vi "Create Message Data Clusters (complex).vi"(8 "error in (no error)":errorcluster, 10 "Message Metadata":T1, 11 "LVClassLibrary in":refnum<vi>) -> (0 "error out":errorcluster, 3 "LVClassLibrary out":refnum<vi>)   [LabVIEW 2019, in "gRPC Scripting Tools.lvlib"]
uses:
  gRPC Scripting Tools.lvlib
  TypeDefs/Message Metadata (Scripting).ctl
  TypeDefs/Message Element Metadata (Scripting).ctl
  gRPC interface/Server API/typeDefs/Message Element Type.ctl
  gRPC interface/gprc-lvsupport.lvlib
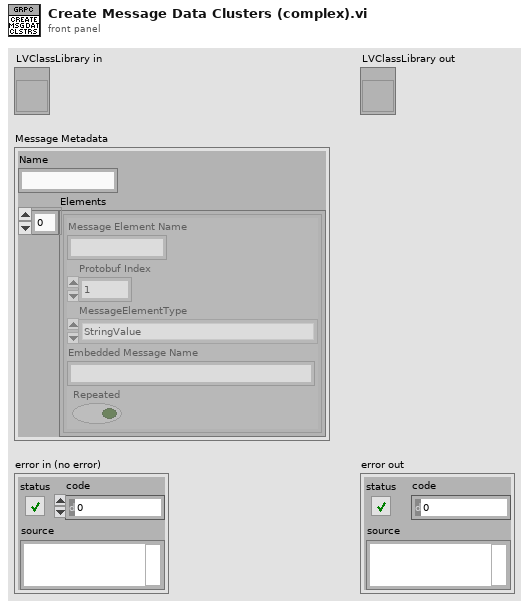
[diagram p1: front panel]
types:
  T1 = typedef "gRPC Scripting Tools.lvlib/Message Metadata (Scripting).ctl" = cluster{"Name":string, "Elements":T2[]}
  T2 = typedef "gRPC Scripting Tools.lvlib/Message Element Metadata (Scripting).ctl" = cluster{"Message Element Name":string, "Protobuf Index":i32, "MessageElementType":T3, "Embedded Message Name":string, "Repeated":bool}
  T3 = typedef "gprc-lvsupport.lvlib/Message Element Type.ctl" = enum32{"Int32Value", "FloatValue", "DoubleValue", "BoolValue", "StringValue", "MessageValue", ""}
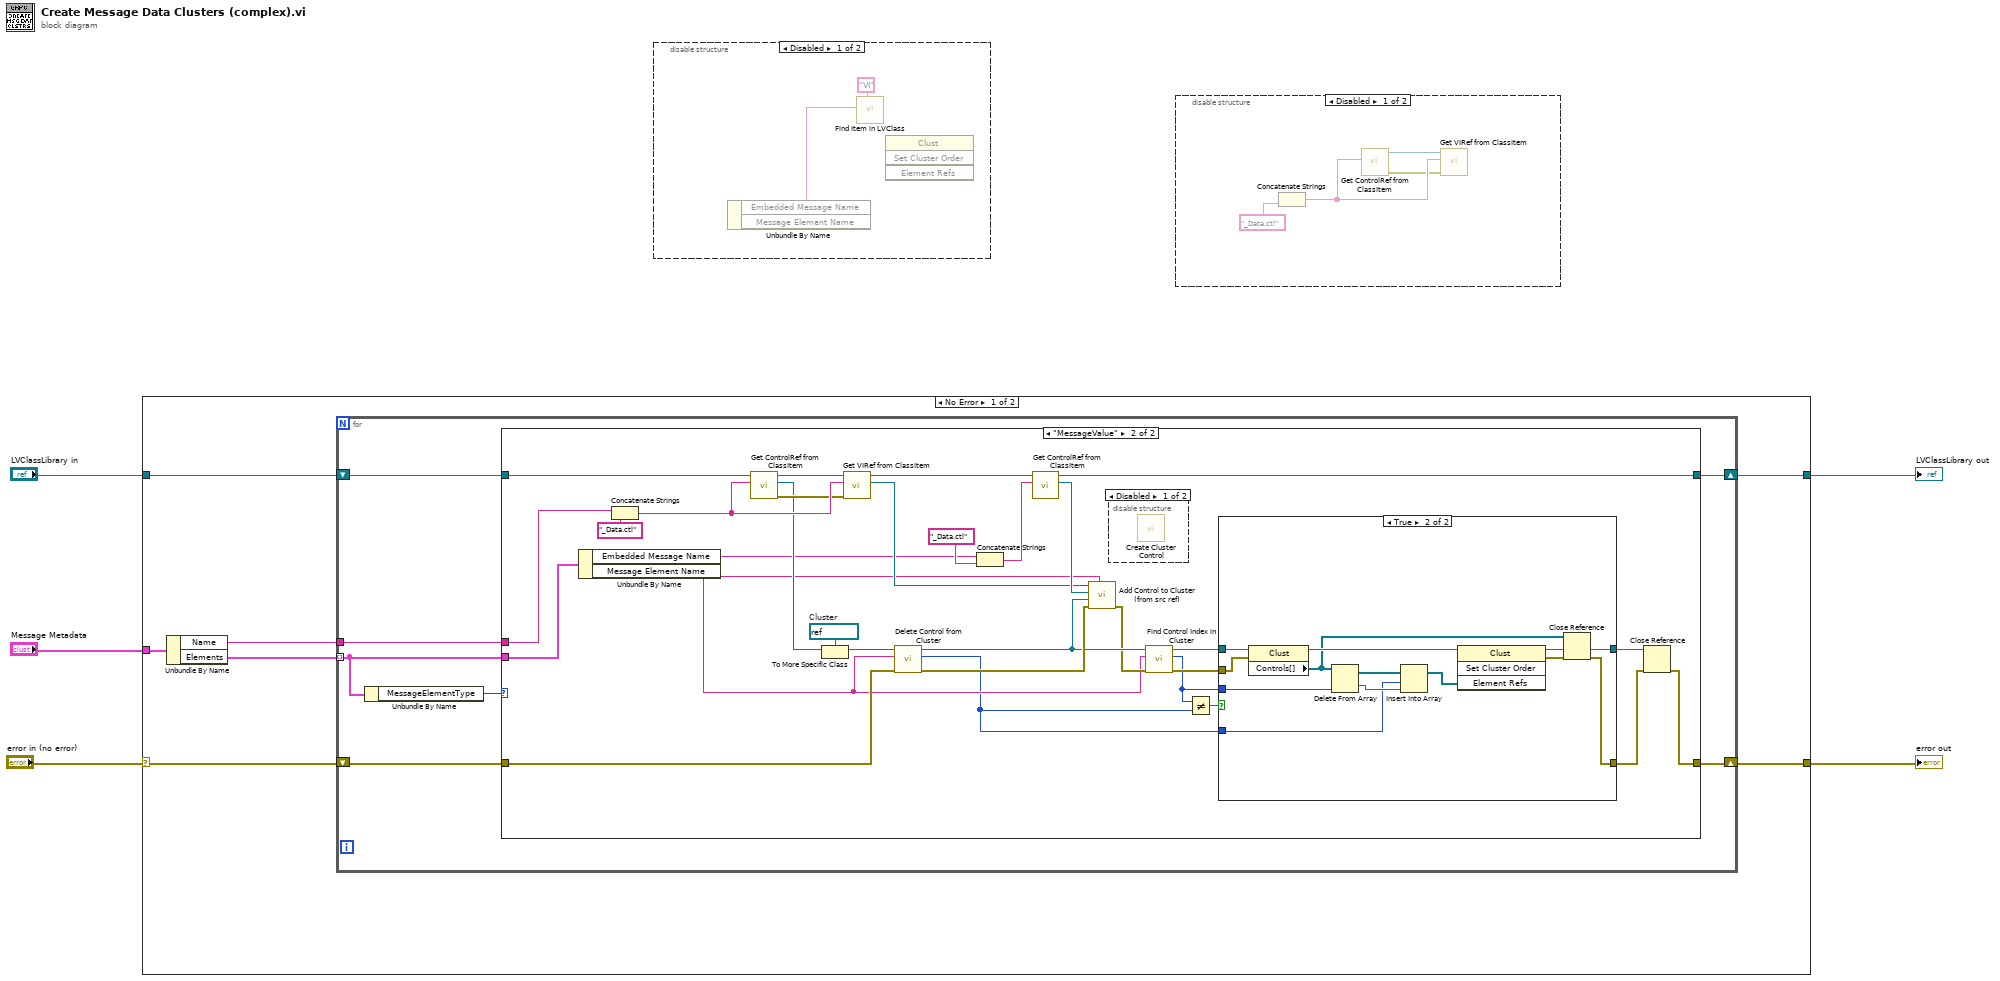
[diagram p0: block diagram]
diagram:
  n1 = case shown="No Error" "error in (no error)" {
    selector: "error in (no error)" -> [w7 w66]
    tunnel: "Message Metadata" -> [w12 _]
    tunnel: "LVClassLibrary in" -> [w8 w67]
    tunnel: [w9 w66] -> w3
    tunnel: [w10 w67] -> w2
    frame No Error {
      n2 = Unbundle By Name(w12) -> ("Name"=w6:string, "Elements"=w11:T2[])
      n3 = for {
        tunnel: w11 -> [w16] mode=indexing
        shift-right: [w17] -> w10
        shift-left: w8 -> [w18]
        shift-right: [w13] -> w9
        shift-left: w7 -> [w14]
        tunnel: w6 -> [w15]
        n4 = Unbundle By Name(w16) -> ("MessageElementType"=w19:T3)
        n5 = case shown="\"MessageValue\"" w19 {
          tunnel: w16 -> [_ w35]
          tunnel: w18 -> [w21 w42]
          tunnel: [w21 w48] -> w17
          tunnel: w15 -> [_ w40]
          tunnel: w14 -> [w20 w33]
          tunnel: [w20 w23] -> w13
          frame "", Default {
          }
          frame "MessageValue" {
            w37 = refnum<vi> refnum  # Cluster
            n6 = Unbundle By Name(w35) -> ("Embedded Message Name"=w34:string, "Message Element Name"=w30:string)
            n7 = Concatenate Strings(w40, "_Data.ctl" ("string")) -> (w44:string)
            n8 = call "Get ControlRef from ClassItem.vi"("Item Name"=w44, "LVClassLibrary in"=w42) -> ("error out"=w43:errorcluster, "Control ref out"=w38:refnum<vi>, "LVClassLibrary out"=w45:refnum<vi>)  [unwired: 6 in, 1 out]
            n9 = To More Specific Class(target class=w37, reference=w38) -> (specific class reference=w36:refnum<vi>)  [unwired: 1 in, 1 out]
            n10 = call "Get VIRef from ClassItem.vi"("error in (no error)"=w43, "Item Name"=w44, "LVClassLibrary in"=w45) -> ("VIref out"=w39:refnum<vi>, "LVClassLibrary out"=w41:refnum<vi>)  [unwired: 5 in, 2 out]
            n11 = call "Delete Control from Cluster.vi"("error in (no error)"=w33, "Control Name in"=w30, "Cluster ref in"=w36) -> ("error out"=w47:errorcluster, "Deleted Index"=w25:i32, "Cluster ref out"=w32:refnum<vi>)  [unwired: 6 in]
            n12 = Concatenate Strings(w34, "_Data.ctl" ("string")) -> (w50:string)
            n13 = call "Get ControlRef from ClassItem.vi"("Item Name"=w50, "LVClassLibrary in"=w41) -> ("Control ref out"=w49:refnum<vi>, "LVClassLibrary out"=w48:refnum<vi>)  [unwired: 6 in, 2 out]
            n14 = call "Add Control to Cluster (from src ref).vi"("New Control Label"=w30, "error in (no error)"=w47, "Cluster ref in (owner)"=w32, "Control ref in"=w49, "Owning VI ref in"=w39) -> ("error out"=w31:errorcluster)  [unwired: 3 in, 3 out]
            n15 = disable-structure shown="Disabled" {
              frame Disabled {
                n16 = call "Create Cluster Control.vi"() -> ()  [unwired: 9 in, 3 out]
              }
              frame Enabled {
              }
            }
            n17 = call "Find Control Index in Cluster.vi"("error in (no error)"=w31, "Control Name"=w30, "Cluster ref in"=w32) -> ("error out"=w27:errorcluster, "Control Index"=w26:i32, "Cluster ref out"=w28:refnum<vi>)  [unwired: 6 in]
            n18 = Not Equal?(x=w26, y=w25) -> (x != y?=w29:bool)
            n19 = case shown="True" w29 {
              tunnel: w28 -> [w52 w65]
              tunnel: w27 -> [w53 w64]
              tunnel: w26 -> [_ w63]
              tunnel: w25 -> [_ w60]
              tunnel: [w53 w55] -> w24
              tunnel: [w52 w54] -> w22
              frame False {
              }
              frame True {
                n20 = property class="Clust"(reference=w65, error in=w64) -> (reference out=w59:refnum<vi>, "Controls[]"=w56:refnum<vi>[])  [unwired: 1 out]
                n21 = Delete From Array(array=w56, index=w63) -> (deleted portion=w61:refnum<vi>, array with subset deleted=w62:refnum<vi>[])  [unwired: 1 in]
                n22 = Insert Into Array(array=w62, index=w60, new element=w61) -> (w58:refnum<vi>[])
                n23 = invoke class="Clust" method="Set Cluster Order"(reference=w59, "Element Refs"=w58) -> (reference out=w54:refnum<vi>, error out=w57:errorcluster)  [unwired: 2 in, 2 out]
                n24 = Close Reference(reference=w56, error in (no error)=w57) -> (error out=w55:errorcluster)
              }
            }
            n25 = Close Reference(reference=w22, error in (no error)=w24) -> (error out=w23:errorcluster)
          }
        }
      }
    }
    frame Error {
    }
  }
  "error out" <- w3
  "LVClassLibrary out" <- w2
  n26 = disable-structure shown="Disabled" {
    frame Disabled {
      n27 = Unbundle By Name() -> ("Embedded Message Name"=w69:string)  [unwired: 1 in, 1 out]
      n28 = call "Find Item in LVClass.vi"("Item Type"="VI", "Item Name"=w69) -> ()  [unwired: 6 in, 4 out]
      n29 = invoke class="Clust" method="Set Cluster Order"() -> ()  [unwired: 4 in, 4 out]
    }
    frame Enabled {
    }
  }
  n30 = disable-structure shown="Disabled" {
    frame Disabled {
      n31 = Concatenate Strings("_Data.ctl" ("string")) -> (w71:string, w75:string)
      n32 = call "Get ControlRef from ClassItem.vi"("Item Name"=w71) -> ("error out"=w70:errorcluster, "Control ref out"=w73:refnum<vi>, "LVClassLibrary out"=w72:refnum<vi>)  [unwired: 7 in, 1 out]
      n33 = call "Get VIRef from ClassItem.vi"("error in (no error)"=w70, "Item Name"=w71, "LVClassLibrary in"=w72) -> ()  [unwired: 5 in, 4 out]
    }
    frame Enabled {
    }
  }
